vi "PROVA WT.vi"() -> ()   [LabVIEW 2019]
panel:
  in  "ID Query (T: Check)":bool=TRUE
  in  "Reset (T: Reset)":bool=TRUE
  in  "STRING":bool
  in  "VISA session (for class)":refnum<visa-resource-name>
  in  "concatenated string":string="TCPIP0::200.0.0.30::10001::SOCKET"
  out "error out 2":errorcluster
  out "error out":errorcluster
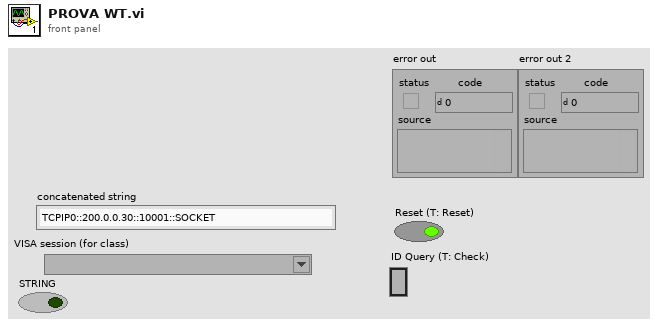
[diagram p1: front panel]
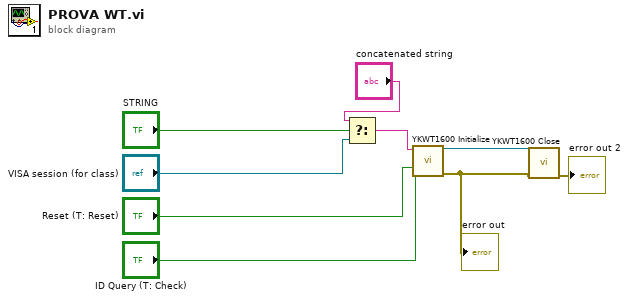
[diagram p0: block diagram]
diagram:
  n1 = Select(t="concatenated string", s="STRING", f="VISA session (for class)") -> (s? t:f=w3:string)
  n2 = call "YKWT1600 Initialize.vi"("VISA session (for class)"=w3, "ID Query (T: Check)"="ID Query (T: Check)", "Reset (T: Reset)"="Reset (T: Reset)") -> ("VISA session"=w8:refnum<visa-resource-name>, "error out"=w7:errorcluster)  [unwired: 11 in]
  "error out" <- w7
  n3 = call "YKWT1600 Close.vi"("VISA session"=w8, "error in (no error)"=w7) -> ("error out"=→"error out 2":errorcluster)  [unwired: 13 in]
